vi "MUX pair error.vi"(8 "error in (no error)":errorcluster, 9 "channel 2":string, 10 "channel 1":string, 11 "SLSC Switch in":refnum<class "SLSC Switch.lvclass">) -> (0 "error out":errorcluster)   [LabVIEW 2016, in "SLSC Switch.lvlib" / "SLSC Switch.lvclass"]
uses:
  SLSC Switch.lvclass
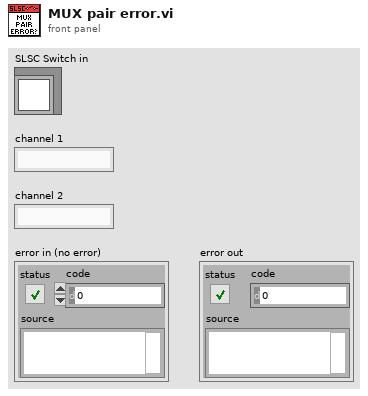
[diagram p1: front panel]
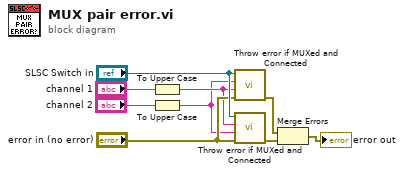
[diagram p0: block diagram]
diagram:
  n1 = To Upper Case(1:"channel 1") -> (0:w3:string)
  n2 = To Upper Case(1:"channel 2") -> (0:w1:string)
  n3 = call "Throw error if MUXed and Connected.vi"("error in (no error)"="error in (no error)", "Destination"=w3, "Source"=w1, "SLSC Switch in"="SLSC Switch in") -> ("error out"=w7:errorcluster)  [unwired: 6 in, 1 out]
  n4 = call "Throw error if MUXed and Connected.vi"("error in (no error)"="error in (no error)", "Destination"=w1, "Source"=w3, "SLSC Switch in"="SLSC Switch in") -> ("error out"=w8:errorcluster)  [unwired: 6 in, 1 out]
  n5 = Merge Errors(w7, w8) -> (→"error out":errorcluster)
